vi "TimeInterpBoolean_GetNewestSample.vi"(11 "TimeInterpBoolean":T1) -> (1 "IsPresent":bool, 2 "TimeStamp":dbl, 3 "OutputBoolean":bool)   [LabVIEW 2019, in "Trajectory_Library.lvlib"]
doc: "Get the newest sample\n\nInputs:\n - TimeInterpBoolean -- Input data cluster\n\nOutputs\n - OutputBoolean -- Newest Boolean. \n - TimeStamp -- Time for this sample (seconds)\n - IsPresent -- Returns TRUE if the buffer contains any data"
uses:
  Trajectory_Library.lvlib
  TypeDef/TIME_INTERPOLATABLE_BOOLEAN.ctl
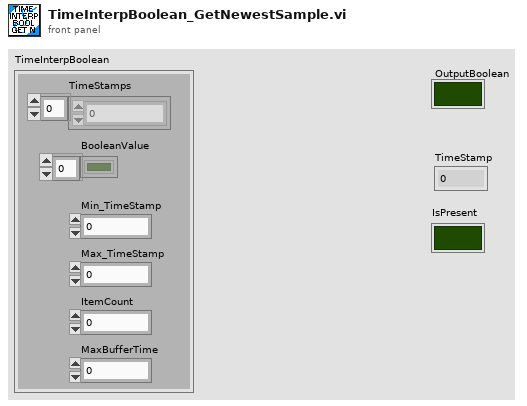
[diagram p1: front panel]
types:
  T1 = typedef "Trajectory_Library.lvlib/TIME_INTERPOLATABLE_BOOLEAN.ctl" = cluster{"TimeStamps":dbl[], "BooleanValue":bool[], "Min_TimeStamp":dbl, "Max_TimeStamp":dbl, "ItemCount":i32, "MaxBufferTime":dbl}
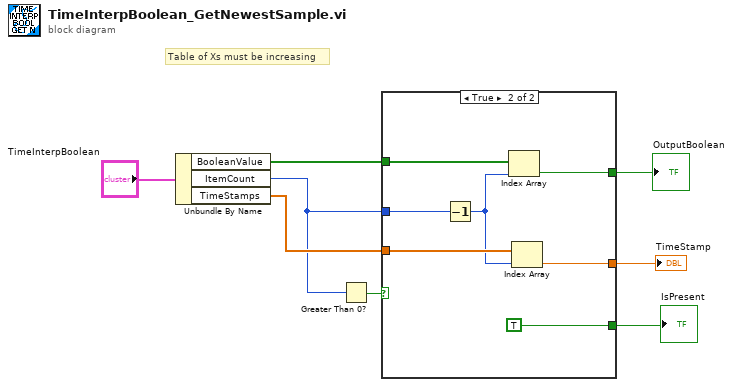
[diagram p0: block diagram]
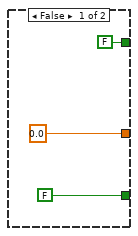
[diagram p2: hidden frame]
diagram:
  # "Table of Xs must be increasing"
  n1 = Unbundle By Name("TimeInterpBoolean") -> ("BooleanValue"=w6:bool[], "ItemCount"=w4:i32, "TimeStamps"=w7:dbl[])
  n2 = Greater Than 0?(x=w4) -> (x > 0?=w5:bool)
  n3 = case shown="True" w5 {
    tunnel: [FALSE ("Table Y") w15] -> w2
    tunnel: w4 -> [_ w13]
    tunnel: w7 -> [_ w17]
    tunnel: w6 -> [_ w18]
    tunnel: [FALSE TRUE] -> w3
    tunnel: [0.0 w16] -> w1
    frame False {
    }
    frame True {
      n4 = Decrement(x=w13) -> (x-1=w12:i32)
      n5 = Index Array(array=w18, index=w12) -> (element=w15:bool)
      n6 = Index Array(array=w17, index=w12) -> (element=w16:dbl)
    }
  }
  "OutputBoolean" <- w2
  "IsPresent" <- w3
  "TimeStamp" <- w1
